vi "PSTR-Plot Response Amplitudes.vi"(0 "Data":T1, 5 "XYGraph":refnum<vi>, 9 "Freq index":i32) -> ()   [LabVIEW 2020]
uses:
  Typedefs/PSTR-Data.ctl
  Typedefs/PSTR-Model Fit.ctl
  Typedefs/PSTR-Fit Parameters.ctl
panel:
  # "NF x NL x 2 x Npts"
  # "NF x NL x Npts"
  # "NF x NL"
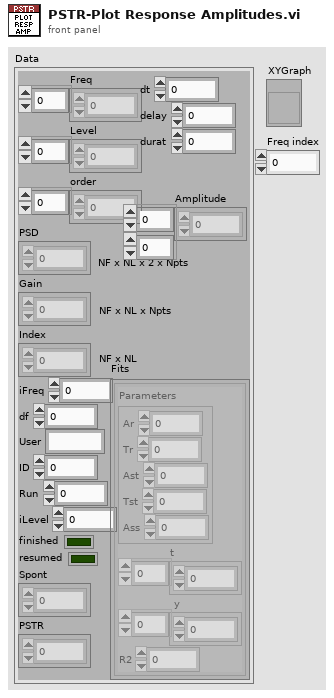
[diagram p1: front panel]
types:
  T1 = typedef "PSTR-Data.ctl" = cluster{"Freq":dbl[], "Level":dbl[], "order":i32[], "PSD":dbl[][][][], "Gain":dbl[][][], "Index":dbl[][], "iFreq":i32, "df":dbl, "User":string, "ID":i32, "Run":i32, "iLevel":i32, "finished":bool, "resumed":bool, "Spont":dbl[][], "PSTR":dbl[][][], "dt":dbl, "delay":dbl, "durat":dbl, "Fits":T2[][], "Amplitude":dbl[][]}
  T2 = typedef "PSTR-Model Fit.ctl" = cluster{"Parameters":T3, "t":dbl[], "y":dbl[], "R2":dbl}
  T3 = typedef "PSTR-Fit Parameters.ctl" = cluster{"Ar":dbl, "Tr":dbl, "Ast":dbl, "Tst":dbl, "Ass":dbl}
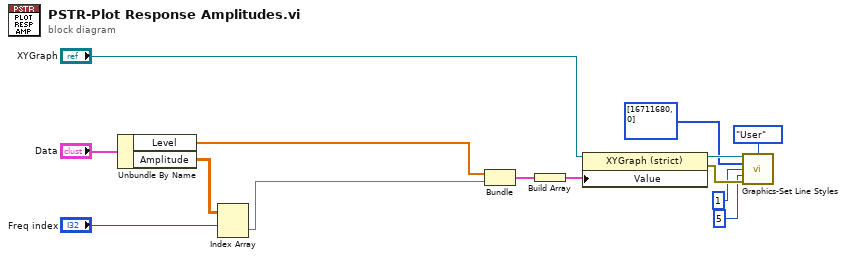
[diagram p0: block diagram]
diagram:
  n1 = Unbundle By Name("Data") -> ("Level"=w4:dbl[], "Amplitude"=w13:dbl[][])
  n2 = Index Array(array=w13, index (row)="Freq index") -> (element=w1:dbl[])  [unwired: 1 in]
  n3 = Bundle("Level"=w4, "Amplitude"=w1) -> (w12:cluster{"Level":dbl[], "Amplitude":dbl[]})  [unwired: 1 in]
  n4 = Build Array(w12) -> (w3:cluster{"Level":dbl[], "Amplitude":dbl[]}[])
  n5 = property class="XYGraph (strict)"(reference="XYGraph", "Value"=w3) -> (reference out=w10:refnum<vi>, error out=w9:errorcluster)  [unwired: 1 in]
  n6 = call "Graphics-Set Line Styles.vi"("XY Graph"=w10, "Map"=enum16{"User", "Prism", "Kelly", "Dark2"}."User", "Colors"=u32[] [16711680, 0], "Plot.Line Width"=u8 1, "Plot.Point Style"=u8 5, "error in (no error)"=w9) -> ()  [unwired: 8 in, 2 out]
